vi "json Member Names.vi"   [LabVIEW 2015, in "JSON Document.lvclass"]
uses:
  JSON Document.lvclass
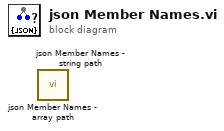
[diagram p0: block diagram]
diagram:
  n1 = call "json Member Names - array path.vi"() -> ()  [unwired: 9 in, 3 out]
  n2 = call "json Member Names - string path.vi"() -> ()  [unwired: 9 in, 3 out]
